vi "test.vi"() -> ()   [LabVIEW 2010]
panel:
  out "path":path
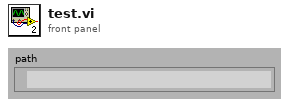
[diagram p1: front panel]
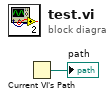
[diagram p0: block diagram]
diagram:
  n1 = Current VI's Path() -> (path=→"path":path)
